vi "叶绿素a校准.vi"() -> ()   [LabVIEW 2016, in "国弘多参数.lvlib"]
uses:
  <vilib>/Utility/miscctls.llb/LVPointTypeDef.ctl
  <vilib>/Analysis/NI_AALBase.lvlib
panel:
  out "温度测量值":dbl caption="温度"
  out "变异系数":dbl
  out "standard deviation":dbl caption="标准差" format="%0.2f"
  out "mean":dbl caption="均值" format="%0.2f"
  out "提示":string
  in  "第一点通过校正":bool
  in  "零点校正":bool
  out "测试值":dbl
  out "电极斜率":dbl
  out "电极零点":dbl
  # "叶绿素a电极设定"
  # "电极校正"
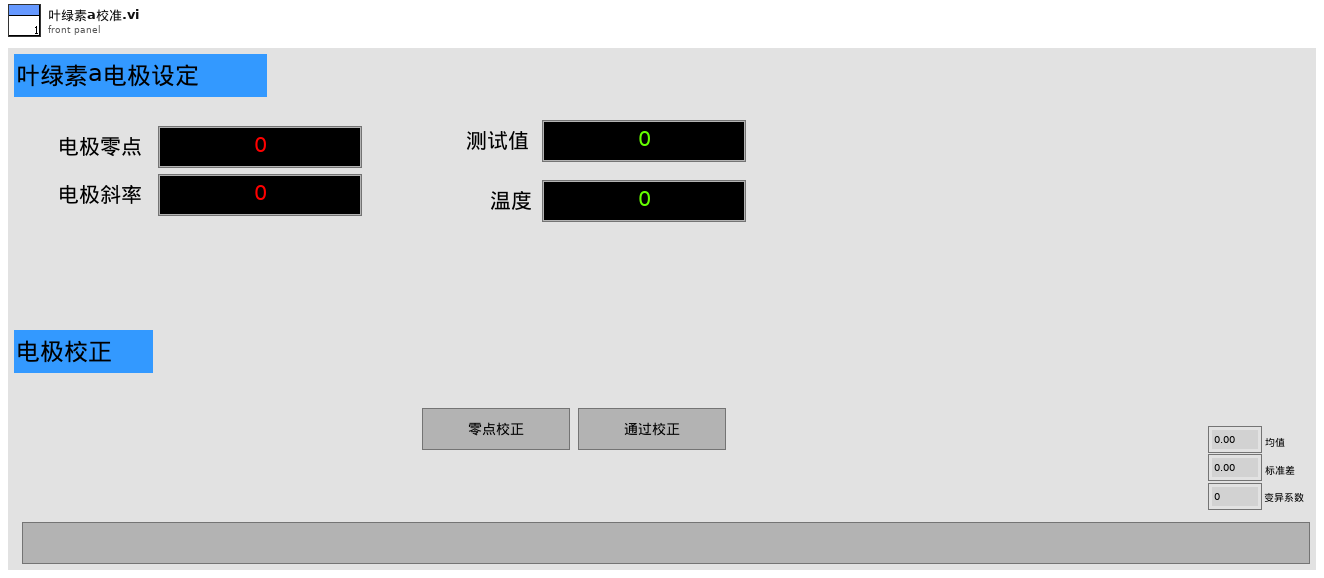
[diagram p1: front panel]
types:
  T1 = typedef "LVPointTypeDef.ctl" = cluster{"Horizontal":i16, "Vertical":i16}
  T2 = typedef "国弘多参数.lvlib/校准步骤.ctl" = enum16{"待机", "第一点校准启动", "第二点校准启动", "第一点校准写入", "第二点校准写入", "第一点校准失败", "第二点校准失败"}
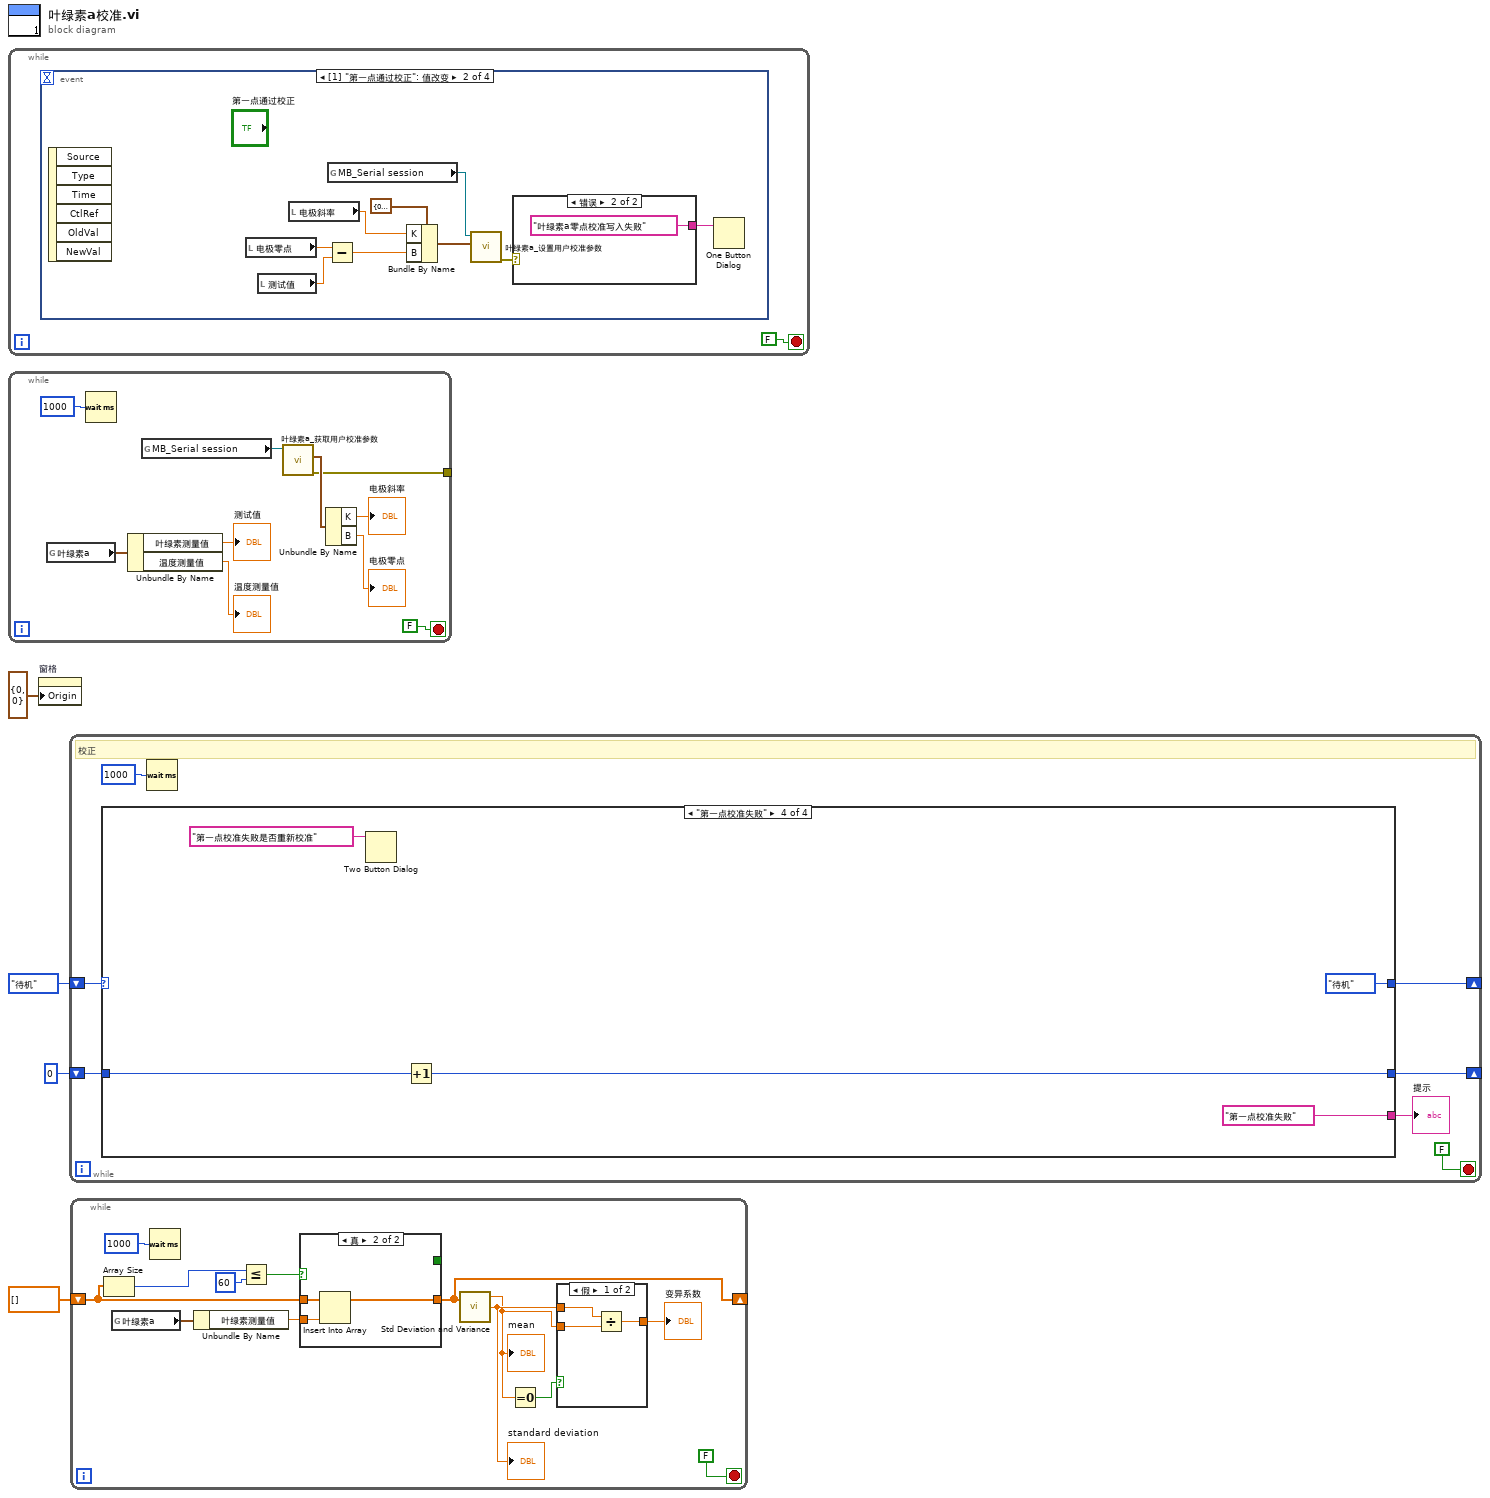
[diagram p0: block diagram]
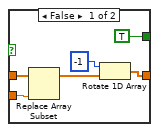
[diagram p3: hidden frame]
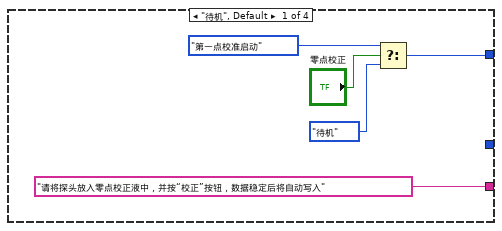
[diagram p4: hidden frame]
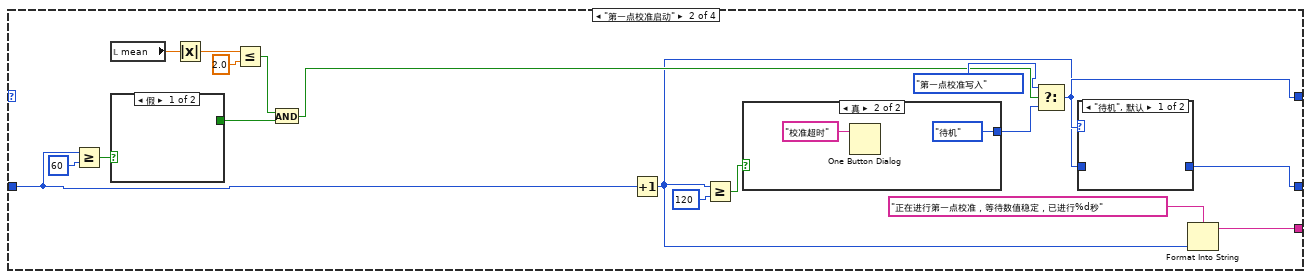
[diagram p5: hidden frame]
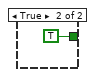
[diagram p6: hidden frame]
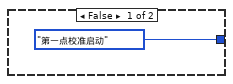
[diagram p8: hidden frame]
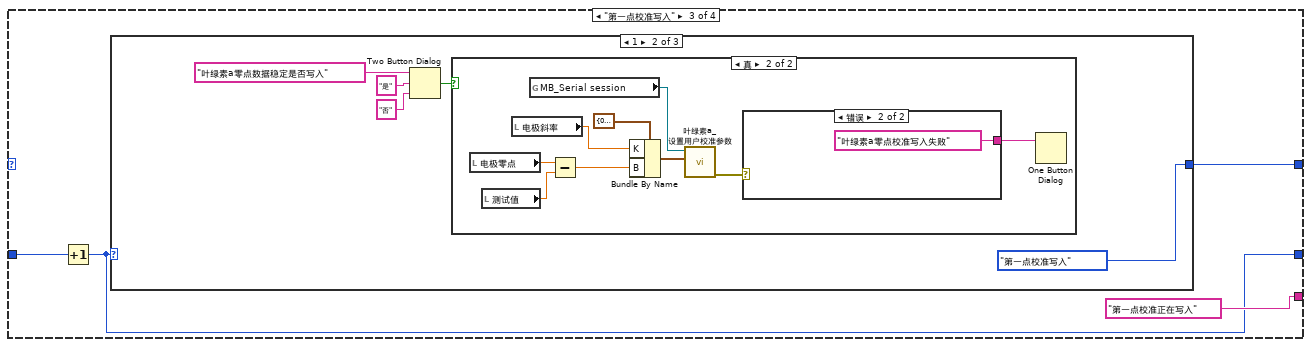
[diagram p9: hidden frame]
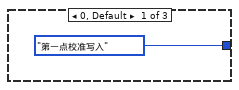
[diagram p10: hidden frame]
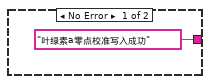
[diagram p12: hidden frame]
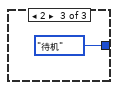
[diagram p13: hidden frame]
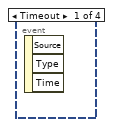
[diagram p14: hidden frame]
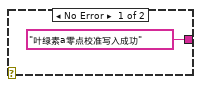
[diagram p15: hidden frame]
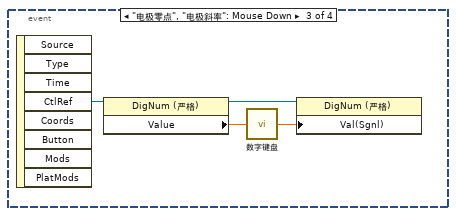
[diagram p16: hidden frame]
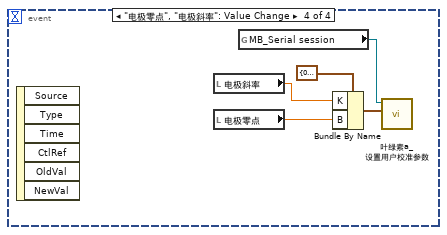
[diagram p17: hidden frame]
diagram:
  n1 = while {
    stop <- FALSE stop-if-true
    n2 = event shown="[1] \"第一点通过校正\": 值改变" {
      selector: _ -> [_ _ _ _]
      dyn-events: _ -> [_ _ _ _]
      timeout: _ -> [_ _ _ _]
      event Timeout {
        n3 = event-data() -> ()  [unwired: 1 in, 3 out]
      }
      event "第一点通过校正": Value Change {
        n4 = event-data() -> ()  [unwired: 1 in, 6 out]
        n5 = local read "电极零点"() -> (w9:dbl)
        n6 = local read "测试值"() -> (w8:dbl)
        n7 = local read "电极斜率"() -> (w10:dbl)
        n8 = Subtract(x=w9, y=w8) -> (x-y=w7:dbl)
        n9 = global read "过程全局变量.vi" "MB_Serial session"() -> (w13:refnum<class "MB_Master_Serial.lvclass">)
        n10 = Bundle By Name(cluster=cluster{"K":sgl, "B":sgl} {"K"=0.0, "B"=0.0} ("用户校准参数"), "K"=w10, "B"=w7) -> (w11:cluster{"K":sgl, "B":sgl})
        n11 = call "叶绿素a_设置用户校准参数.vi"("用户校准参数"=w11, "MB_Serial session in"=w13) -> ("error out"=w6:errorcluster)  [unwired: 8 in, 1 out]
        n12 = case shown="错误" w6 {
          tunnel: ["叶绿素a零点校准写入成功" ("消息") "叶绿素a零点校准写入失败" ("消息")] -> w14
          frame No Error {
          }
          frame Error {
          }
        }
        n13 = One Button Dialog(message=w14) -> ()  [unwired: 1 in, 1 out]
      }
      event "电极零点", "电极斜率": Mouse Down {
        n14 = event-data() -> ("CtlRef"=w17:refnum<vi>)  [unwired: 1 in, 7 out]
        n15 = property class="DigNum (严格)"(reference=w17) -> (reference out=w18:refnum<vi>, "Value"=w19:dbl)  [unwired: 1 in, 1 out]
        n16 = call "数字键盘.vi"("OldNumber"=w19) -> ("NewNumber"=w20:sgl)
        n17 = property class="DigNum (严格)"(reference=w18, "Val(Sgnl)"=w20) -> ()  [unwired: 1 in, 2 out]
      }
      event "电极零点", "电极斜率": Value Change {
        n18 = event-data() -> ()  [unwired: 1 in, 6 out]
        n19 = local read "电极斜率"() -> (w22:dbl)
        n20 = local read "电极零点"() -> (w21:dbl)
        n21 = global read "过程全局变量.vi" "MB_Serial session"() -> (w25:refnum<class "MB_Master_Serial.lvclass">)
        n22 = Bundle By Name(cluster=cluster{"K":sgl, "B":sgl} {"K"=0.0, "B"=0.0} ("用户校准参数"), "K"=w22, "B"=w21) -> (w23:cluster{"K":sgl, "B":sgl})
        n23 = call "叶绿素a_设置用户校准参数.vi"("用户校准参数"=w23, "MB_Serial session in"=w25) -> ()  [unwired: 8 in, 2 out]
      }
    }
  }
  n24 = while {
    tunnel: [w29] -> _
    stop <- FALSE stop-if-true
    n25 = global read "过程全局变量.vi" "叶绿素a"() -> (w28:cluster{"温度测量值":sgl, "叶绿素测量值":sgl, "错误标志":u16})
    n26 = Wait (ms)(milliseconds to wait=u32 1000 ("等待时间（毫秒）")) -> ()  [unwired: 1 out]
    n27 = Unbundle By Name(w28) -> ("叶绿素测量值"=→"测试值":sgl, "温度测量值"=→"温度测量值":sgl)
    n28 = global read "过程全局变量.vi" "MB_Serial session"() -> (w33:refnum<class "MB_Master_Serial.lvclass">)
    n29 = call "叶绿素a_获取用户校准参数.vi"("MB_Serial session in"=w33) -> ("error out"=w29:errorcluster, "输出值"=w32:cluster{"K":sgl, "B":sgl})  [unwired: 8 in, 1 out]
    n30 = Unbundle By Name(w32) -> ("K"=→"电极斜率":sgl, "B"=→"电极零点":sgl)
  }
  n31 = property on="窗格" class="Pane"("Origin"=T1 {"Horizontal"=0, "Vertical"=0} ("原点")) -> ()  [unwired: 2 in, 2 out]
  n32 = while "While循环" {
    shift-right: [w41] -> _
    shift-left: 校准步骤."待机" ("枚举") -> [w42]
    shift-right: [w37] -> _
    shift-left: 0 -> [w38]
    stop <- FALSE stop-if-true
    # "校正"
    n33 = case shown="\"第一点校准失败\"" w42 {
      tunnel: [w46 w55 w71 校准步骤."待机" ("枚举")] -> w41
      tunnel: ["请将探头放入零点校正液中，并按“校正”按钮，数据稳定后将自动写入" ("提示") w64 "第一点校准正在写入" ("提示") "第一点校准失败" ("提示")] -> w36
      tunnel: w38 -> [_ w50 w73 w94]
      tunnel: [_ w53 w72 w93] -> w37
      frame "待机", Default {
        n34 = Select(t=校准步骤."第一点校准启动" ("枚举"), s="零点校正", f=校准步骤."待机" ("枚举")) -> (s? t:f=w46:T2)
      }
      frame "第一点校准启动" {
        n35 = Greater Or Equal?(x=w50, y=60) -> (x >= y?=w51:bool)
        n36 = local read "mean"() -> (w48:dbl)
        n37 = case shown="假" w51 {
          tunnel: [_ TRUE] -> w49
          frame False {
          }
          frame True {
          }
        }
        n38 = Absolute Value(x=w48) -> (abs(x)=w59:dbl)
        n39 = Less Or Equal?(x=w59, y=2.0) -> (x <= y?=w61:bool)
        n40 = And(x=w61, y=w49) -> (x .and. y?=w60:bool)
        n41 = Increment(x=w50) -> (x+1=w54:i32)
        n42 = Greater Or Equal?(x=w54, y=120) -> (x >= y?=w57:bool)
        n43 = case shown="真" w57 {
          tunnel: [校准步骤."第一点校准启动" ("枚举") 校准步骤."待机" ("枚举")] -> w56
          frame False {
          }
          frame True {
            n44 = One Button Dialog(message="校准超时" ("消息")) -> ()  [unwired: 1 in, 1 out]
          }
        }
        n45 = Select(t=校准步骤."第一点校准写入" ("枚举"), s=w60, f=w56) -> (s? t:f=w55:T2)
        n46 = case shown="\"待机\", 默认" w55 {
          tunnel: w54 -> [_ w67]
          tunnel: [_ w67] -> w53
          frame "待机", Default {
          }
          frame "第一点校准启动" {
          }
        }
        n47 = Format Into String(format string="正在进行第一点校准，等待数值稳定，已进行%d秒" ("格式字符串"), w54) -> (resulting string=w64:string)  [unwired: 2 in, 1 out]
      }
      frame "第一点校准写入" {
        n48 = Increment(x=w73) -> (x+1=w72:i32)
        n49 = case shown="1" w72 {
          tunnel: [校准步骤."第一点校准写入" ("枚举") 校准步骤."第一点校准写入" ("枚举") 校准步骤."待机" ("枚举")] -> w71
          frame 0, Default {
          }
          frame 1 {
            n50 = Two Button Dialog(message="叶绿素a零点数据稳定是否写入" ("消息"), 1:"否" ("F按钮名称（“取消”）"), 2:"是" ("T按钮名称（“确定”）")) -> (T button?=w76:bool)
            n51 = case shown="真" w76 {
              frame False {
              }
              frame True {
                n52 = local read "电极零点"() -> (w84:dbl)
                n53 = local read "测试值"() -> (w83:dbl)
                n54 = local read "电极斜率"() -> (w85:dbl)
                n55 = global read "过程全局变量.vi" "MB_Serial session"() -> (w88:refnum<class "MB_Master_Serial.lvclass">)
                n56 = Subtract(x=w84, y=w83) -> (x-y=w82:dbl)
                n57 = Bundle By Name(cluster=cluster{"K":sgl, "B":sgl} {"K"=0.0, "B"=0.0} ("用户校准参数"), "K"=w85, "B"=w82) -> (w86:cluster{"K":sgl, "B":sgl})
                n58 = call "叶绿素a_设置用户校准参数.vi"("用户校准参数"=w86, "MB_Serial session in"=w88) -> ("error out"=w81:errorcluster)  [unwired: 8 in, 1 out]
                n59 = case shown="错误" w81 {
                  tunnel: ["叶绿素a零点校准写入成功" ("消息") "叶绿素a零点校准写入失败" ("消息")] -> w89
                  frame No Error {
                  }
                  frame Error {
                  }
                }
                n60 = One Button Dialog(message=w89) -> ()  [unwired: 1 in, 1 out]
              }
            }
          }
          frame 2 {
          }
        }
      }
      frame "第一点校准失败" {
        n61 = Two Button Dialog(message="第一点校准失败是否重新校准" ("消息")) -> ()  [unwired: 2 in, 1 out]
        n62 = Increment(x=w94) -> (x+1=w93:i32)
      }
    }
    "提示" <- w36
    n63 = Wait (ms)(milliseconds to wait=u32 1000 ("等待时间（毫秒）")) -> ()  [unwired: 1 out]
  }
  n64 = while {
    shift-right: [w103] -> _
    shift-left: sgl[] [] -> [w106]
    stop <- FALSE stop-if-true
    n65 = Array Size(array=w106) -> (size(s)=w108:i32)
    n66 = global read "过程全局变量.vi" "叶绿素a"() -> (w100:cluster{"温度测量值":sgl, "叶绿素测量值":sgl, "错误标志":u16})
    n67 = Wait (ms)(milliseconds to wait=u32 1000 ("等待时间（毫秒）")) -> ()  [unwired: 1 out]
    n68 = Unbundle By Name(w100) -> ("叶绿素测量值"=w105:sgl)
    n69 = Less Or Equal?(x=w108, y=60) -> (x <= y?=w107:bool)
    n70 = case shown="真" w107 {
      tunnel: w106 -> [w119 w122]
      tunnel: w105 -> [w117 w121]
      tunnel: [w115 w120] -> w103
      tunnel: [TRUE _] -> _
      frame False {
        n71 = Replace Array Subset(array=w119, new element=w117) -> (w118:sgl[])  [unwired: 1 in]
        n72 = Rotate 1D Array(1:w118, 2:-1 ("n")) -> (0:w115:sgl[])
      }
      frame True {
        n73 = Insert Into Array(array=w122, new element=w121) -> (w120:sgl[])  [unwired: 1 in]
      }
    }
    n74 = call <vilib>:"Std Deviation and Variance.vi"("X"=w103) -> ("mean"=w98:dbl, "standard deviation"=w99:dbl)  [unwired: 1 in, 1 out]
    "standard deviation" <- w99
    "mean" <- w98
    n75 = Equal To 0?(x=w98) -> (x = 0?=w104:bool)
    n76 = case shown="假" w104 {
      tunnel: w99 -> [w113 _]
      tunnel: [w112 _] -> w102
      tunnel: w98 -> [w111 _]
      frame False {
        n77 = Divide(x=w113, y=w111) -> (x/y=w112:dbl)
      }
      frame True {
      }
    }
    "变异系数" <- w102
  }
